vi "GetGObjectCoordinates__slk_mt.vi"(6 "bounds type (Master)":enum16{"Master", "Total"}(ring), 8 "error in (no error)":errorcluster, 11 "generic objects refnums in":refnum<vi>[](array[refnum])) -> (0 "error out":errorcluster, 1 "bounds":cluster{"Width":u32, "Height":u32}, 2 "position":cluster{"Left":i32, "Top":i32}, 3 "rectangle":T1)   [LabVIEW 2020, in "Lazyboots Menu Tool.lvlib"]
doc: "Returns the rectangle, position and bounds of a group of objects."
uses:
  Library/Lazyboots Menu Tool.lvlib
panel:
  # "GetGObjectCoordinates__slk_mt.vi\nReturns the rectangle, position and bounds of a group of objects.\n\nNOTICE -- YOU MUST LEAVE THIS NOTICE IN PLACE.\n\nCopyright (c) 2011, LIANG LIU Shawn.Liu.cn@gmail.com\nAll rights reserved.\n\nRedistribution and use in source and binary forms, with or without modification, are permitted provided that the following conditions are met:\n-Redistributions of source code must retain the above copyright notice, this list of conditions and the following disclaimer.\n-Redistributions in binary form must reproduce the above copyright notice, this list of conditions and the following disclaimer in the documentation and/or other materials provided with the distribution.\n-Neither the name of the eLp nor the names of its contributors may be used to endorse or promote products derived from this software without specific prior written permission.\n\nTHIS SOFTWARE IS PROVIDED BY THE COPYRIGHT HOLDERS AND CONTRIBUTORS \"AS IS\" AND ANY EXPRESS OR IMPLIED WARRANTIES, INCLUDING, BUT NOT LIMITED TO, THE IMPLIED WARRANTIES OF MERCHANTABILITY AND FITNESS FOR A PARTICULAR PURPOSE ARE DISCLAIMED. IN NO EVENT SHALL THE COPYRIGHT HOLDER OR CONTRIBUTORS BE LIABLE FOR ANY DIRECT, INDIRECT, INCIDENTAL, SPECIAL, EXEMPLARY, OR CONSEQUENTIAL DAMAGES (INCLUDING, BUT NOT LIMITED TO, PROCUREMENT OF SUBSTITUTE GOODS OR SERVICES; LOSS OF USE, DATA, OR PROFITS; OR BUSINESS INTERRUPTION) HOWEVER CAUSED AND ON ANY THEORY OF LIABILITY, WHETHER IN CONTRACT, STRICT LIABILITY, OR TORT (INCLUDING NEGLIGENCE OR OTHERWISE) ARISING IN ANY WAY OUT OF THE USE OF THIS SOFTWARE, EVEN IF ADVISED OF THE POSSIBILITY OF SUCH DAMAGE."
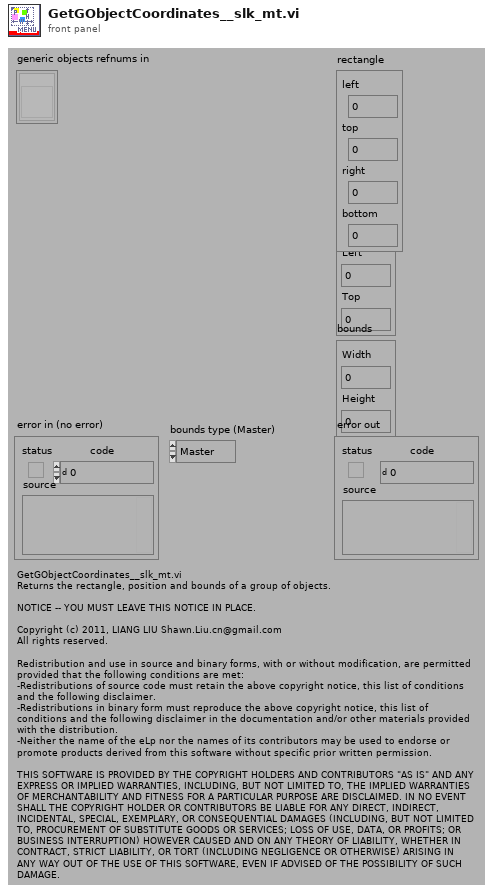
[diagram p1: front panel]
types:
  T1 = cluster{"left":i16, "top":i16, "right":i16, "bottom":i16}
  T2 = typedef "LVRectTypeDef.ctl" = cluster{"Left":i16, "Top":i16, "Right":i16, "Bottom":i16}
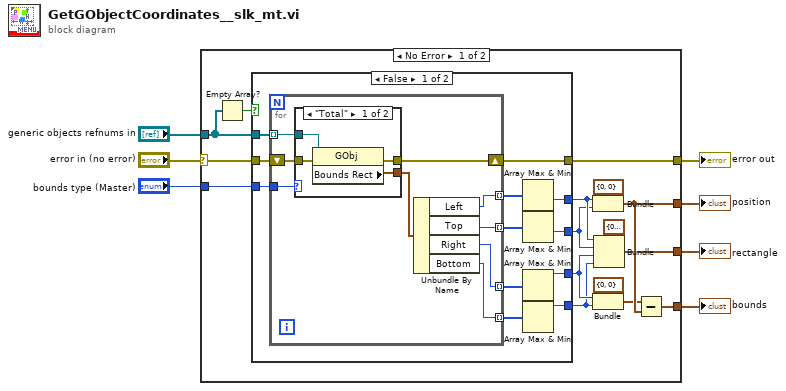
[diagram p0: block diagram]
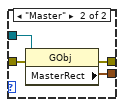
[diagram p2: hidden frame]
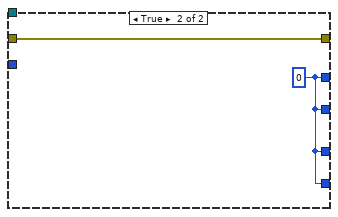
[diagram p3: hidden frame]
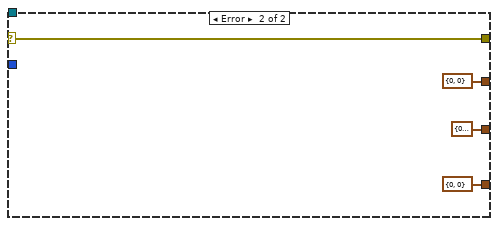
[diagram p4: hidden frame]
diagram:
  n1 = case shown="No Error" "error in (no error)" {
    selector: "error in (no error)" -> [w19 w58]
    tunnel: [w23 w58] -> w7
    tunnel: [w22 cluster{u32, u32} {0, 0}] -> w6
    tunnel: [w21 cluster{"Left":i32, "Top":i32} {"Left"=0, "Top"=0} ("position")] -> w5
    tunnel: [w20 T1 {"left"=0, "top"=0, "right"=0, "bottom"=0} ("total rectangle")] -> w4
    tunnel: "generic objects refnums in" -> [w18 _]
    tunnel: "bounds type (Master)" -> [w8 _]
    frame No Error {
      n2 = Empty Array?(array=w18) -> (empty?=w9:bool)
      n3 = case shown="False" w9 {
        tunnel: [w35 w54] -> w23
        tunnel: w19 -> [w34 w54]
        tunnel: w18 -> [w33 _]
        tunnel: [w28 w53] -> w13
        tunnel: [w27 w53] -> w12
        tunnel: [w26 w53] -> w11
        tunnel: [w25 w53] -> w10
        tunnel: w8 -> [w24 _]
        frame False {
          n4 = for {
            tunnel: w33 -> [w37] mode=indexing
            tunnel: [w41] -> w30 mode=indexing
            tunnel: [w40] -> w31 mode=indexing
            tunnel: [w39] -> w32 mode=indexing
            shift-right: [w43] -> w35
            shift-left: w34 -> [w44]
            tunnel: [w38] -> w29 mode=indexing
            tunnel: w24 -> [w36]
            n5 = case shown="\"Total\"" w36 {
              tunnel: w44 -> [w48 w52]
              tunnel: [w47 w51] -> w43
              tunnel: [w46 w50] -> w42
              tunnel: w37 -> [w45 w49]
              frame "Total" {
                n6 = property class="GObj"(reference=w45, error in=w48) -> (error out=w47:errorcluster, "Bounds Rect"=w46:T2)  [unwired: 1 out]
              }
              frame "Master" {
                n7 = property class="GObj"(reference=w49, error in=w52) -> (error out=w51:errorcluster, "MasterRect"=w50:T2)  [unwired: 1 out]
              }
            }
            n8 = Unbundle By Name(w42) -> ("Left"=w41:i16, "Top"=w40:i16, "Right"=w39:i16, "Bottom"=w38:i16)
          }
          n9 = Array Max & Min(array=w30) -> (min value=w28:i16)  [unwired: 3 out]
          n10 = Array Max & Min(array=w31) -> (min value=w27:i16)  [unwired: 3 out]
          n11 = Array Max & Min(array=w32) -> (max value=w26:i16)  [unwired: 3 out]
          n12 = Array Max & Min(array=w29) -> (max value=w25:i16)  [unwired: 3 out]
        }
        frame True {
          w53 = i16 0 ("left")
          (unwired) i16 0
        }
      }
      n13 = Bundle(cluster=cluster{"Left":i32, "Top":i32} {"Left"=0, "Top"=0} ("position"), "Left"=w13, "Top"=w12) -> (w21:cluster{"Left":i32, "Top":i32})
      n14 = Bundle(cluster=cluster{"Width":u32, "Height":u32} {"Width"=0, "Height"=0} ("bounds"), "Width"=w11, "Height"=w10) -> (w17:cluster{"Width":u32, "Height":u32})
      n15 = Bundle(cluster=T1 {"left"=0, "top"=0, "right"=0, "bottom"=0} ("total rectangle"), "left"=w13, "top"=w12, "right"=w11, "bottom"=w10) -> (w20:T1)
      n16 = Subtract(x=w17, y=w21) -> (x-y=w22:cluster{u32, u32})
    }
    frame Error {
    }
  }
  "position" <- w5
  "bounds" <- w6
  "error out" <- w7
  "rectangle" <- w4
